vi "MT Detect Offset PSK.vi"(5 "input complex waveform":T3={"t0"=0.0, "dt"=1.0, "Y"=[]} {"Y" format="%.3f"; "dt" format="%^.2e"; "t0" format="%.4f"}, 7 "Offset PSK system parameters":T2={"samples per symbol (16)"=16, "symbol map"=[], "differential Offset PSK"=enum."disable"} {"symbol map" format="%.3f"}, 9 "synchronization parameters":T1 {"sync sequence" format="%.2f"}, 11 "error in (no error)":errorcluster, 12 "matched filter coefficients":dbl[](array[numeric]) format="%.2f", 13 "reset? (T)":bool=TRUE, 14 "flush buffers? (F)":bool) -> (6 "output bit stream":i8[](array[numeric]), 10 "sync found index (symbols)":dbl format="%.4f", 15 "error out":errorcluster)   [LabVIEW 2020, in "niDMT.lvlib"]
doc: "Demodulates a offset PSK-modulated complex baseband waveform and returns the demodulated bit stream. This VI attempts to remove carrier and phase offset by locking to the carrier signal."
uses:
  <vilib>/addons/Modulation/niDMT.lvlib
  <vilib>/addons/Modulation/Analog/controls/Complex Data Waveform.ctl
  <vilib>/addons/Modulation/Digital/Support/Controls/Offset PSK System Parameters.ctl
  <vilib>/Utility/error.llb/Error Cluster From Error Code.vi
  <vilib>/addons/Modulation/Digital/Support/Common/mod_Truncate FIR Filter (complex).vi
  <vilib>/addons/Modulation/niAMT.lvlib
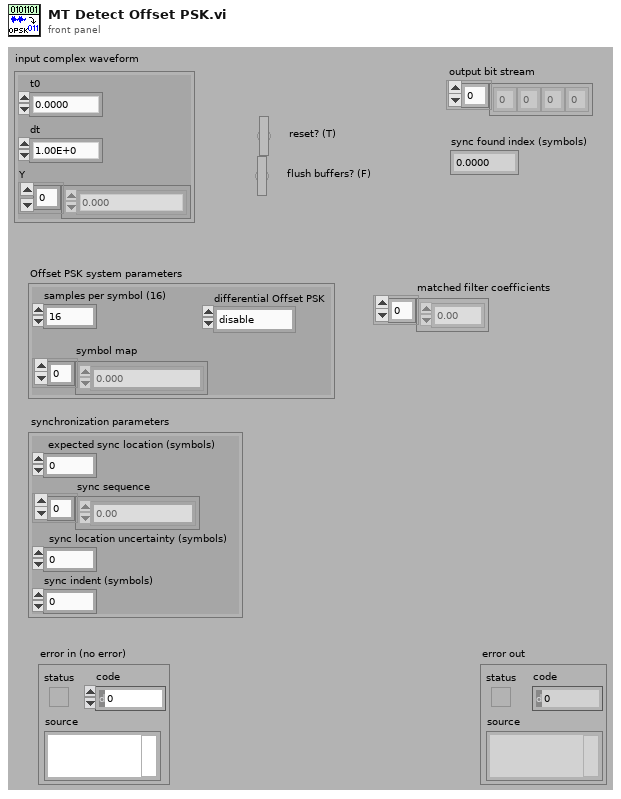
[diagram p1: front panel]
types:
  T1 = cluster{"expected sync location (symbols)":i32, "sync sequence":cdb[], "sync location uncertainty (symbols)":i32, "sync indent (symbols)":i32}
  T2 = typedef "niDMT.lvlib/Offset PSK System Parameters.ctl" = cluster{"samples per symbol (16)":i32, "symbol map":cdb[], "differential Offset PSK":enum16{"disable", "enable"}}
  T3 = typedef "niAMT.lvlib/Complex Data Waveform.ctl" = cluster{"t0":dbl, "dt":dbl, "Y":cdb[]}
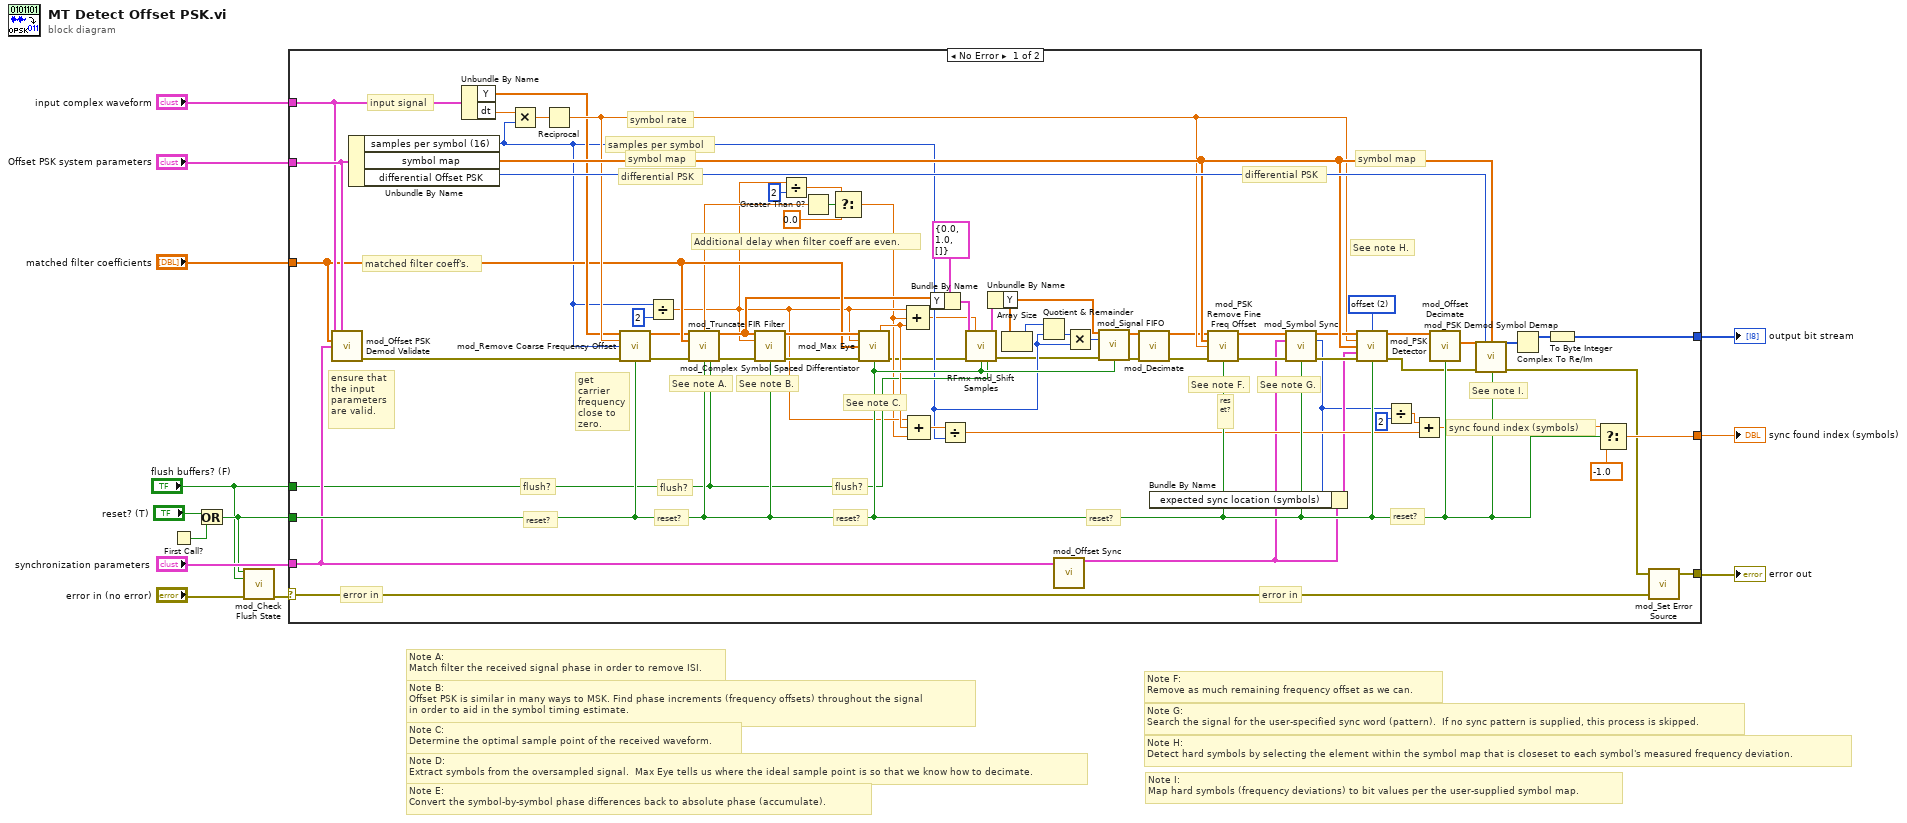
[diagram p0: block diagram]
diagram:
  # "Note E:\nConvert the symbol-by-symbol phase differences back to absolute phase (accumulate)."
  # "Note B:\nOffset PSK is similar in many ways to MSK. Find phase increments (frequency offsets) throughout the signal\nin order to aid in the symbol timing estimate."
  # "Note I:\nMap hard symbols (frequency deviations) to bit values per the user-supplied symbol map."
  # "Note G:\nSearch the signal for the user-specified sync word (pattern).  If no sync pattern is supplied, this process is skipped."
  # "Note F:\nRemove as much remaining frequency offset as we can."
  # "Note D:\nExtract symbols from the oversampled signal.  Max Eye tells us where the ideal sample point is so that we know how to decimate."
  # "Note C:\nDetermine the optimal sample point of the received waveform."
  # "Note A:\nMatch filter the received signal phase in order to remove ISI."
  # "Note H:\nDetect hard symbols by selecting the element within the symbol map that is closeset to each symbol's measured frequency deviation."
  n1 = First Call?() -> (First Call?: T/F=w6:bool)
  n2 = Or(x="reset? (T)", y=w6) -> (x .or. y?=w3:bool)
  n3 = call <vilib>:"mod_Check Flush State.vi"("reset?"=w3, "flush buffers? (F)"="flush buffers? (F)", "error in (no error)"="error in (no error)") -> ("error out"=w4:errorcluster)  [unwired: 12 out]
  n4 = case shown="No Error" w4 {
    selector: w4 -> [w70 w81]
    tunnel: w3 -> [w76 _]
    tunnel: "input complex waveform" -> [w73 _]
    tunnel: [w71 w81] -> w12
    tunnel: "matched filter coefficients" -> [w38 _]
    tunnel: [w80 _] -> w7
    tunnel: [w78 _] -> w10
    tunnel: "Offset PSK system parameters" -> [w74 _]
    tunnel: "synchronization parameters" -> [w72 _]
    tunnel: "flush buffers? (F)" -> [w37 _]
    frame No Error {
      w35 = u16 2 items=["normal", "shifted", "offset"] ("PSK type")
      # "Additional delay when filter coeff are even."
      # "See note I."
      # "flush?"
      # "flush?"
      # "flush?"
      # "reset?"
      # "reset?"
      # "reset?"
      # "symbol map"
      # "symbol map"
      # "matched filter coeff's."
      # "input signal"
      # "symbol rate"
      # "differential PSK"
      # "differential PSK"
      # "samples per symbol"
      # "reset?"
      # "sync found index (symbols)"
      # "reset?"
      # "reset?"
      # "error in"
      # "error in"
      # "error in"
      # "See note H."
      # "See note G."
      # "ensure that the input parameters are valid."
      # "See note A."
      # "See note B."
      # "get carrier frequency close to zero."
      # "See note C."
      # "See note F."
      n5 = call <vilib>:"mod_Offset PSK Demod Validate.vi"("Input Complex Waveform"=w73, "PSK System Parameters"=w74, "Matched Filter Coefficients"=w38, "Synchronization Parameters"=w72) -> ("error out"=w75:errorcluster)  [unwired: 11 out]
      n6 = Unbundle By Name(w74) -> ("samples per symbol (16)"=w26:i32, "symbol map"=w77:cdb[], "differential Offset PSK"=w79:enum16{"disable", "enable"})
      n7 = Unbundle By Name(w73) -> ("Y"=w50:cdb[], "dt"=w67:dbl)
      n8 = Multiply(x=w67, y=w26) -> (x*y=w69:dbl)
      n9 = Reciprocal(x=w69) -> (1/x=w59:dbl)
      n10 = call <vilib>:"mod_Remove Coarse Frequency Offset.vi"("Signal In"=w50, "Symbol Rate, Hz"=w59, "Samples Per Symbol (16)"=w26, "error in (no error)"=w75, "Reset? (T)"=w76) -> ("Signal Out"=w36:cdb[], "error out"=w53:errorcluster)  [unwired: 9 out]
      n11 = Divide(x=w26, y=2) -> (x/y=w30:dbl)
      n12 = call-poly <vilib>:"mod_Truncate FIR Filter.vi"("Signal In"=w36, "Filter Coefficients"=w38, "error in (no error)"=w53, "Reset? (T)"=w76, "flush buffers? (F)"=w37) -> ("Fractional Delay (samples)"=w31:dbl, "Signal Out"=w34:cdb[], "error out"=w52:errorcluster)  [unwired: 8 out]
      n13 = call <vilib>:"mod_Complex Symbol Spaced Differentiator.vi"("Signal In"=w34, "Samples Per Symbol (16)"=w30, "error in (no error)"=w52, "Reset? (T)"=w76) -> ("Signal Out"=w49:cdb[], "error out"=w60:errorcluster)  [unwired: 10 out]
      n14 = Divide(x=w30, y=2) -> (x/y=w28:dbl)
      n15 = Greater Than 0?(x=w31) -> (x > 0?=w33:bool)
      n16 = Select(t=w28, s=w33, f=0.0) -> (s? t:f=w27:dbl)
      n17 = call <vilib>:"mod_Max Eye.vi"("Signal In"=w49, "Samples Per Symbol (16)"=w30, "Filter Coefficients"=w38, "error in (no error)"=w60, "Reset? (T)"=w76) -> ("Waveform Alignment Offset"=w46:dbl, "error out"=w22:errorcluster)  [unwired: 6 in, 3 out]
      n18 = Compound Arithmetic op=ADD(w30, w27, w46) -> (w23:dbl)
      n19 = Compound Arithmetic op=ADD(w30, w46, w27) -> (w51:dbl)
      n20 = Bundle By Name(cluster=T3 {"t0"=0.0, "dt"=1.0, "Y"=[]} ("Input Complex Waveform"), "Y"=w34) -> (w24:T3)
      n21 = Divide(x=w51, y=w26) -> (x/y=w68:dbl)
      n22 = call <vilib>:"RFmx mod_Shift Samples.vi"("Input Complex Waveform"=w24, "Initial Sample Offset, sec"=w23, "error in (no error)"=w22, "Reset? (T)"=w76, "flush buffers? (F)"=w37) -> ("Output Complex Waveform"=w21:T3, "error out"=w16:errorcluster)  [unwired: 9 in]
      n23 = Unbundle By Name(w21) -> ("Y"=w18:cdb[])
      n24 = Array Size(array=w18) -> (size(s)=w19:i32)
      n25 = Quotient & Remainder(x=w19, y=w26) -> (floor(x/y)=w20:i32)  [unwired: 1 out]
      n26 = call <vilib>:"mod_Offset Sync.vi"("synchronization parameters in"=w72) -> ("synchronization parameters out"=w58:T1)  [unwired: 14 out]
      n27 = Multiply(x=w20, y=w26) -> (x*y=w17:i32)
      n28 = call <vilib>:"mod_Signal FIFO.vi"("Signal In"=w18, "Output Length"=w17, "error in (no error)"=w16, "Reset? (T)"=w76) -> ("Signal Out"=w15:cdb[], "error out"=w14:errorcluster)  [unwired: 10 out]
      n29 = call <vilib>:"mod_Decimate.vi"("Signal In"=w15, "error in (no error)"=w14) -> ("Signal Out"=w48:cdb[], "error out"=w62:errorcluster)  [unwired: 3 in, 9 out]
      n30 = call <vilib>:"mod_PSK Remove Fine Freq Offset.vi"("Symbols"=w48, "Symbol Map"=w77, "Symbol Rate, Hz"=w59, "error in (no error)"=w62, "Reset? (T)"=w76) -> ("Symbols"=w47:cdb[], "error out"=w65:errorcluster)  [unwired: 9 out]
      n31 = call <vilib>:"mod_Symbol Sync.vi"("Signal In"=w47, "Synchronization Parameters"=w58, "error in (no error)"=w65, "Reset? (T)"=w76) -> ("Signal Out"=w64:cdb[], "Sync Location (symbols)"=w56:i32, "error out"=w63:errorcluster)  [unwired: 9 out]
      n32 = Bundle By Name(cluster=w58, "expected sync location (symbols)"=w56) -> (w61:T1)
      n33 = call <vilib>:"mod_PSK Detector.vi"("Signal In"=w64, "PSK type"=w35, "Symbol Rate, Hz"=w59, "Symbol Map"=w77, "Synchronization Parameters"=w61, "error in (no error)"=w63, "Reset (T)"=w76) -> ("Signal Out"=w57:cdb[], "error out"=w40:errorcluster)  [unwired: 7 out]
      n34 = Divide(x=w56, y=2) -> (x/y=w54:dbl)
      n35 = Add(x=w54, y=w68) -> (x+y=w44:dbl)
      n36 = call <vilib>:"mod_Offset Decimate.vi"("Symbols In"=w57, "Reset (T)"=w76) -> ("Symbols Out"=w41:cdb[])  [unwired: 13 out]
      n37 = call <vilib>:"mod_PSK Demod Symbol Demap.vi"("Symbols In"=w41, "Differential PSK Enable"=w79, "Symbol Map"=w77, "error in (no error)"=w40, "Reset? (T)"=w76) -> ("Bits Out"=w42:i8[], "error out"=w39:errorcluster)  [unwired: 9 out]
      n38 = Complex To Re/Im(x + iy=w42) -> (x=w43:i8[])  [unwired: 1 out]
      n39 = To Byte Integer(number=w43) -> (8bit integer=w80:i8[])
      n40 = Select(t=w44, s=w76, f=-1.0) -> (s? t:f=w78:dbl)
      n41 = call <vilib>:"mod_Set Error Source.vi"("initial error in (no error)"=w70, "final error in (no error)"=w39) -> ("error out"=w71:errorcluster)  [unwired: 3 out]
    }
    frame Error {
    }
  }
  "error out" <- w12
  "sync found index (symbols)" <- w10
  "output bit stream" <- w7
